vi "get_current_position.vi"(0 "reference (in)":i32, 5 "error in (no error)":errorcluster) -> (14 "reference (dup)":i32, 16 "current_position (units)":i32, 19 "error out":errorcluster)   [LabVIEW 2012]
doc: "This VI reads the current position of the motor.\n\nProduced By:\n\nChristopher Lemieux\nKod Integrations, LLC\n4835 Marianne Drive\nMount Airy, MD 21771\nhttp://www.kodintegrations.com\nemail: clemieux@kodintegrations.com\nphone: (240) 687-1288"
uses:
  main_functions/commands.ctl
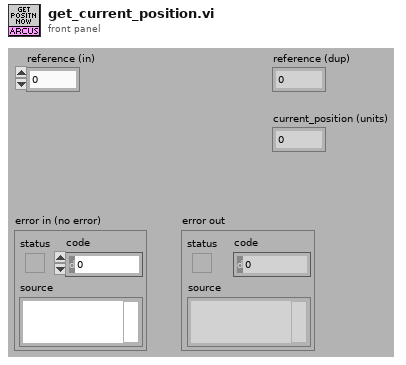
[diagram p1: front panel]
types:
  T1 = typedef "commands.ctl" = enum16{"clear error", "constant jog(-)", "constant jog(+)", "get acceleration", "get actual current", "get device id", "get digital input status", "get digial inputs status", "get dig output status", "get digital outputs status", "get firmware ver", "get high speed", "get idle current", "get low speed", "get micro step", "get motor status", "get move mode", "get polarity", "get position", "get product id", "get power status", "get run current", "get status", "home(-)", "home(+)", "move to position", "power down", "power up", "set acceleration", "set device id", "set digital output", "set digital outputs", "set high speed", "set idle current", "set low speed", "set move mode absolute", "set move mode increment", "set polarity", "set position", "set run current", "stop immediate", "stop slow", "store to memory"}
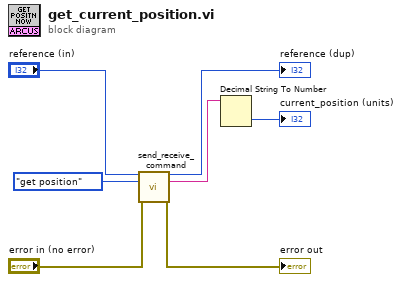
[diagram p0: block diagram]
diagram:
  n1 = call "send_receive_command.vi"("reference (in)"="reference (in)", "command"=commands."get position", "error in (no error)"="error in (no error)") -> ("reference (dup)"=→"reference (dup)":i32, "read_string"=w4:string, "error out"=→"error out":errorcluster)  [unwired: 8 in, 2 out]
  n2 = Decimal String To Number(string=w4) -> (number=→"current_position (units)":i32)  [unwired: 2 in, 1 out]
